vi "Single Digitizer Register Enable.vi"(8 "error in":errorcluster, 9 "Enable":i32 format="%.0x", 10 "Digitizer":i32(ring) items=["Digitizer 1", "Digitizer 2"], 11 "Instrument Handle In":i32) -> (0 "error out":errorcluster, 3 "Instrument Handle Out":i32)   [LabVIEW 8.6, in "ZTScopeM.lvlib"]
doc: "Configure the event forwarding state of the selected digitizer register."
uses:
  ZTScopeM.lvlib
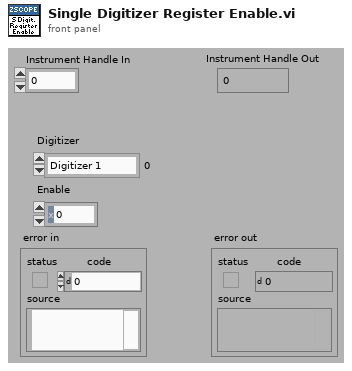
[diagram p1: front panel]
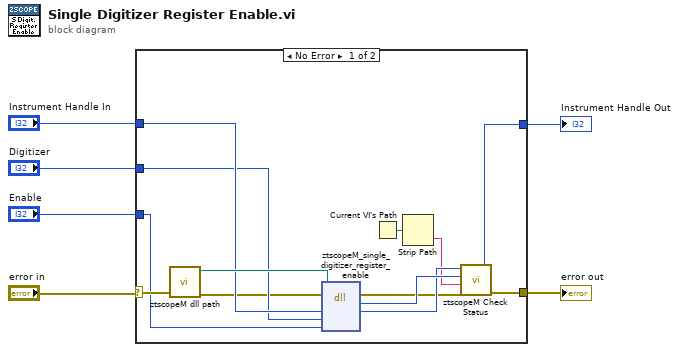
[diagram p0: block diagram]
diagram:
  n1 = case shown="No Error" "error in" {
    selector: "error in" -> [w13 w21]
    tunnel: [w14 w21] -> w5
    tunnel: [w15 w20] -> w4
    tunnel: "Instrument Handle In" -> [w11 w20]
    tunnel: "Digitizer" -> [w10 _]
    tunnel: "Enable" -> [w9 _]
    frame #0 {
      n2 = call "ztscopeM dll path.vi"("error in (no error)"=w13) -> ("error out"=w8:errorcluster, "<instrument>.dll path"=w12:path)  [unwired: 9 in]
      n3 = dll-call lib="C:/Program Files (x86)/National Instruments/LabVIEW 2013/instr.lib/ztscopem/ztscopeM.dll" fn="ztscopeM_single_digitizer_register_enable"(path in=w12, error in=w8, "instrumentHandle"=w11, "cursor"=w10, "enable"=w9) -> (error out=w7:errorcluster, w19:i32, "instrumentHandle"=w18:i32)  [unwired: 3 in, 1 out]
      n4 = Current VI's Path() -> (path=w17:path)
      n5 = Strip Path(path=w17) -> (name=w16:string)  [unwired: 1 out]
      n6 = call "ztscopeM Check Status.vi"("error in"=w7, "name of VI"=w16, "status (return code)"=w19, "instrument handle in"=w18) -> ("error out"=w14:errorcluster, "instrument handle out"=w15:i32)  [unwired: 2 out]
    }
    frame #1 {
    }
  }
  "Instrument Handle Out" <- w4
  "error out" <- w5
